vi "TestExec.Send Funct RTN Data.vi"(8 "Error":errorcluster, 9 "RTN Route (Data2)":variant, 10 "RTN Data":T1 {"MeasData"."Status" items=["LOG", "PASS", "FAIL", "ERROR"]; "Attr"."Status" items=["LOG", "PASS", "FAIL", "ERROR"]; "Num"."Status" items=["LOG", "PASS", "FAIL", "ERROR"]}, 11 "Q In":refnum<queue>) -> (0 "error out":errorcluster)   [LabVIEW 2018]
uses:
  <vilib>/KATE/Queues/Q.Element.ctl
  TestExec.Local Result Data.ctl
  Results/Result.Attribute.ctl
  Results/Result.Measurement and Attribute Item Status.ctl
  Results/Result.Numeric.ctl
  Results/Result.Limit Type.ctl
  Results/Result XML/TestResult.SW Item.ctl
  Reports/Report.Result FileDataObject.ctl
  Results/Result.Measurement Item.ctl
  <vilib>/KATE/Queues/Queue Utils.lvlib
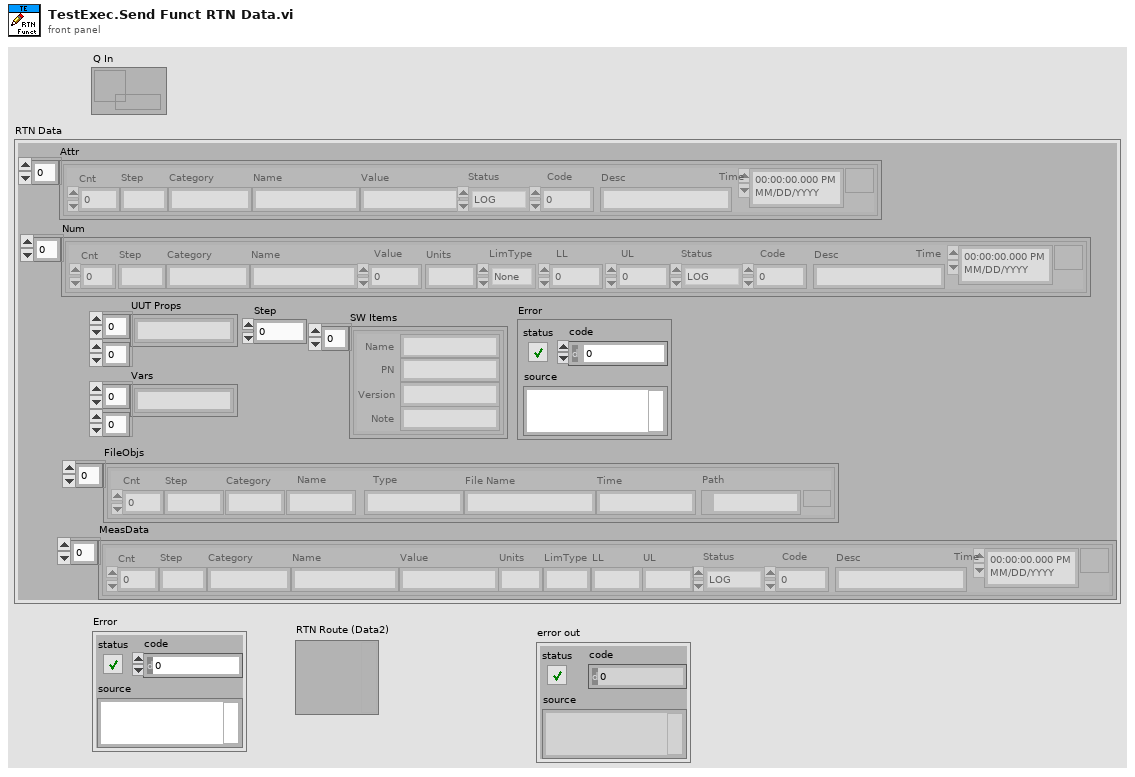
[diagram p1: front panel]
types:
  T1 = typedef "TestExec.Local Result Data.ctl" = cluster{"Attr":T2[], "Num":T4[], "UUT Props":string[][], "Vars":string[][], "SW Items":T6[], "Error":errorcluster, "Step":i32, "FileObjs":T7[], "MeasData":T8[]}
  T2 = typedef "Result.Attribute.ctl" = cluster{"Cnt":i32, "Step":string, "Category":string, "Name":string, "Value":string, "Status":T3, "Code":i32, "Desc":string, "Time":timestamp}
  T3 = typedef "Result.Measurement and Attribute Item Status.ctl" = i32
  T4 = typedef "Result.Numeric.ctl" = cluster{"Cnt":i32, "Step":string, "Category":string, "Name":string, "Value":dbl, "Units":string, "LimType":T5, "LL":dbl, "UL":dbl, "Status":T3, "Code":i32, "Desc":string, "Time":timestamp}
  T5 = typedef "Result.Limit Type.ctl" = enum16{"None", "EQ", "NE", "GT", "LT", "GE", "LE", "GTLT", "GELE", "GELT", "GTLE", "LTGT", "LEGE", "LEGT", "LTGE", "Contains", "NotContains"}
  T6 = typedef "TestResult.SW Item.ctl" = cluster{"Name":string, "PN":string, "Version":string, "Note":string}
  T7 = typedef "Report.Result FileDataObject.ctl" = cluster{"Cnt":i32, "Step":string, "Category":string, "Name":string, "Type":string, "File Name":string, "Time":string, "Path":path}
  T8 = typedef "Result.Measurement Item.ctl" = cluster{"Cnt":i32, "Step":string, "Category":string, "Name":string, "Value":string, "Units":string, "LimType":string, "LL":string, "UL":string, "Status":T3, "Code":i32, "Desc":string, "Time":timestamp}
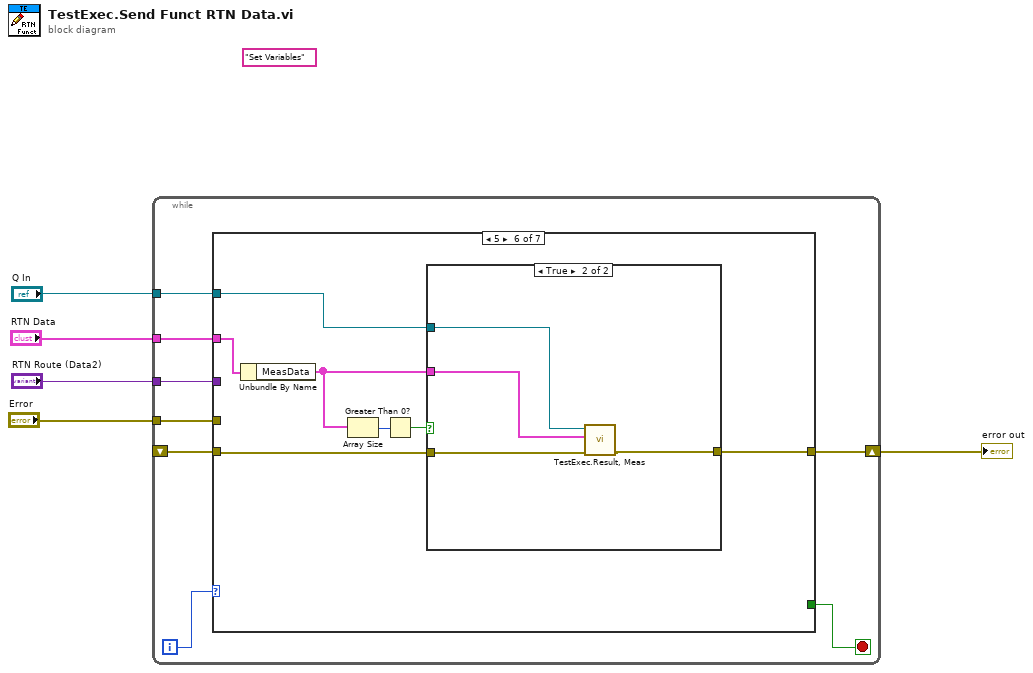
[diagram p0: block diagram]
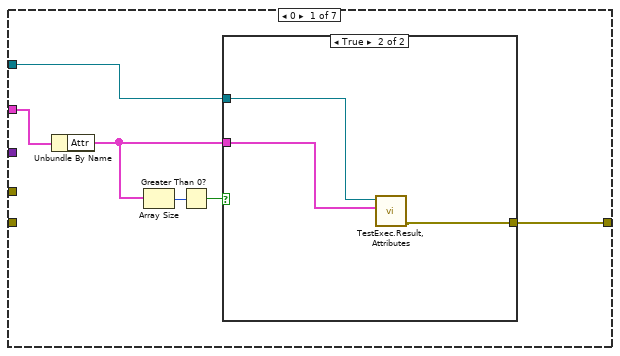
[diagram p2: hidden frame]
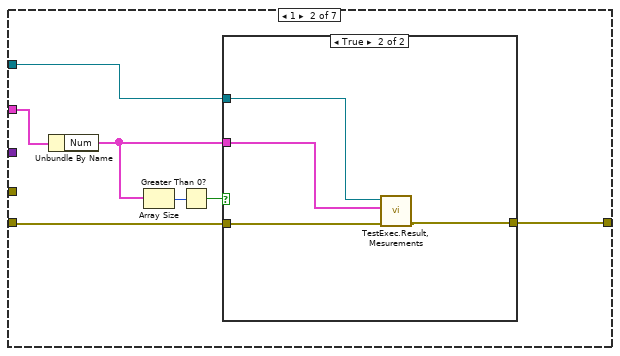
[diagram p4: hidden frame]
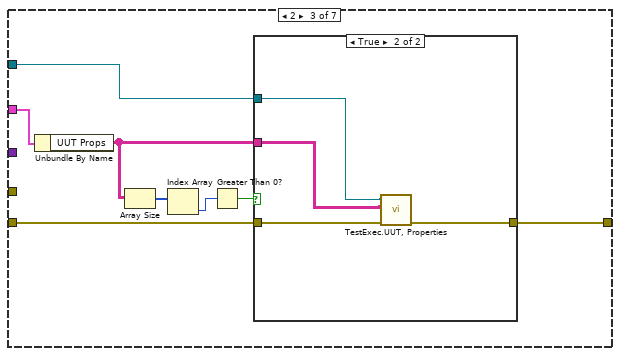
[diagram p6: hidden frame]
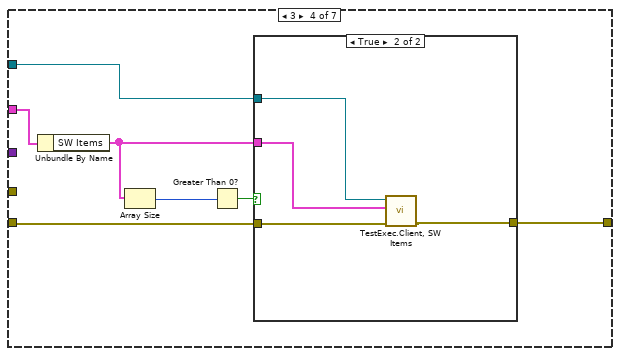
[diagram p8: hidden frame]
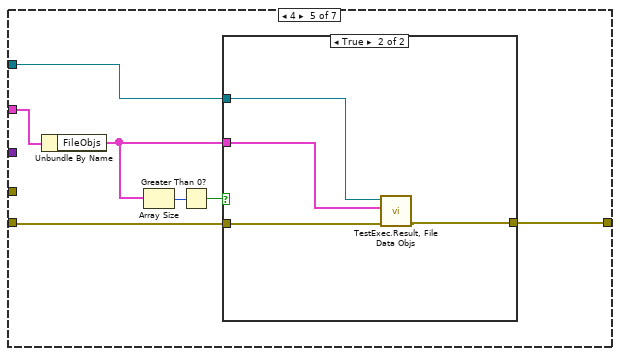
[diagram p10: hidden frame]
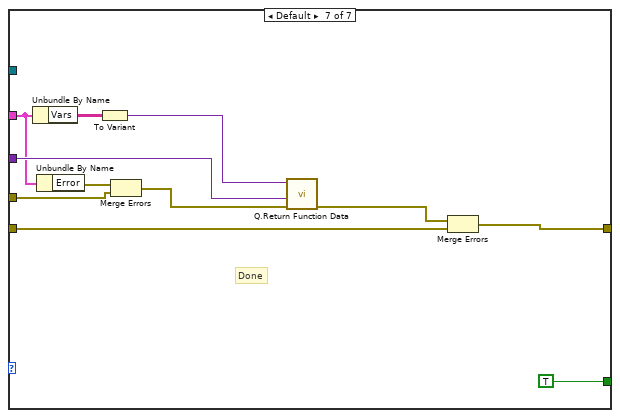
[diagram p13: hidden frame]
diagram:
  (unwired) "Set Variables" ("Cmd")
  n1 = while {
    shift-right: [w10] -> w5
    shift-left: _ -> [w11]
    tunnel: "RTN Data" -> [w9]
    tunnel: "Q In" -> [w8]
    tunnel: "RTN Route (Data2)" -> [w7]
    tunnel: "Error" -> [w6]
    i -> [w13]
    stop <- w12 stop-if-true
    n2 = case shown="5" w13 {
      tunnel: [_ _ _ _ _ _ TRUE] -> w12
      tunnel: w11 -> [_ w23 w34 w46 w57 w68 w84]
      tunnel: [w15 w25 w38 w49 w59 w70 w83] -> w10
      tunnel: w9 -> [w19 w29 w41 w52 w63 w74 w82]
      tunnel: w8 -> [w14 w24 w37 w48 w58 w69 _]
      tunnel: w7 -> [_ _ _ _ _ _ w88]
      tunnel: w6 -> [_ _ _ _ _ _ w80]
      frame 0 {
        n3 = Unbundle By Name(w19) -> ("Attr"=w16:T2[])
        n4 = Array Size(array=w16) -> (size(s)=w17:i32)
        n5 = Greater Than 0?(x=w17) -> (x > 0?=w18:bool)
        n6 = case shown="True" w18 {
          tunnel: w16 -> [_ w21]
          tunnel: [_ w20] -> w15
          tunnel: w14 -> [_ w22]
          frame False {
          }
          frame True {
            n7 = call "TestExec.Result, Attributes.vi"("Attributes"=w21, "Q In"=w22) -> ("error out"=w20:errorcluster)  [unwired: 9 in]
          }
        }
      }
      frame 1 {
        n8 = Unbundle By Name(w29) -> ("Num"=w26:T4[])
        n9 = Array Size(array=w26) -> (size(s)=w27:i32)
        n10 = Greater Than 0?(x=w27) -> (x > 0?=w28:bool)
        n11 = case shown="True" w28 {
          tunnel: w26 -> [_ w32]
          tunnel: [_ w31] -> w25
          tunnel: w24 -> [_ w33]
          tunnel: w23 -> [_ w30]
          frame False {
          }
          frame True {
            n12 = call "TestExec.Result, Mesurements.vi"("error in"=w30, "Measurements"=w32, "Q In"=w33) -> ("error out"=w31:errorcluster)  [unwired: 8 in]
          }
        }
      }
      frame 2 {
        n13 = Unbundle By Name(w41) -> ("UUT Props"=w39:string[][])
        n14 = Array Size(array=w39) -> (size(s)=w36:i32[])
        n15 = Index Array(array=w36) -> (element=w35:i32)  [unwired: 1 in]
        n16 = Greater Than 0?(x=w35) -> (x > 0?=w40:bool)
        n17 = case shown="True" w40 {
          tunnel: w39 -> [_ w44]
          tunnel: [_ w43] -> w38
          tunnel: w37 -> [_ w45]
          tunnel: w34 -> [_ w42]
          frame False {
          }
          frame True {
            n18 = call "TestExec.UUT, Properties.vi"("error in"=w42, "UUT Properties"=w44, "Q In"=w45) -> ("error out"=w43:errorcluster)  [unwired: 8 in]
          }
        }
      }
      frame 3 {
        n19 = Unbundle By Name(w52) -> ("SW Items"=w50:T6[])
        n20 = Array Size(array=w50) -> (size(s)=w47:i32)
        n21 = Greater Than 0?(x=w47) -> (x > 0?=w51:bool)
        n22 = case shown="True" w51 {
          tunnel: w50 -> [_ w54]
          tunnel: [_ w55] -> w49
          tunnel: w48 -> [_ w56]
          tunnel: w46 -> [_ w53]
          frame False {
          }
          frame True {
            n23 = call "TestExec.Client, SW Items.vi"("error in"=w53, "SW Items"=w54, "Q In"=w56) -> ("error out"=w55:errorcluster)  [unwired: 7 in, 1 out]
          }
        }
      }
      frame 4 {
        n24 = Unbundle By Name(w63) -> ("FileObjs"=w60:T7[])
        n25 = Array Size(array=w60) -> (size(s)=w61:i32)
        n26 = Greater Than 0?(x=w61) -> (x > 0?=w62:bool)
        n27 = case shown="True" w62 {
          tunnel: w60 -> [_ w66]
          tunnel: [_ w65] -> w59
          tunnel: w58 -> [_ w67]
          tunnel: w57 -> [_ w64]
          frame False {
          }
          frame True {
            n28 = call "TestExec.Result, File Data Objs.vi"("error in"=w64, "File Data Objs"=w66, "Q In"=w67) -> ("error out"=w65:errorcluster)  [unwired: 8 in]
          }
        }
      }
      frame 5 {
        n29 = Unbundle By Name(w74) -> ("MeasData"=w71:T8[])
        n30 = Array Size(array=w71) -> (size(s)=w72:i32)
        n31 = Greater Than 0?(x=w72) -> (x > 0?=w73:bool)
        n32 = case shown="True" w73 {
          tunnel: w71 -> [_ w77]
          tunnel: [_ w76] -> w70
          tunnel: w69 -> [_ w78]
          tunnel: w68 -> [_ w75]
          frame False {
          }
          frame True {
            n33 = call "TestExec.Result, Meas.vi"("error in"=w75, "Meas"=w77, "Q In"=w78) -> ("error out"=w76:errorcluster)  [unwired: 8 in]
          }
        }
      }
      frame Default {
        # "Done"
        n34 = Unbundle By Name(w82) -> ("Vars"=w87:string[][])
        n35 = Unbundle By Name(w82) -> ("Error"=w81:errorcluster)
        n36 = To Variant(anything=w87) -> (Variant=w86:variant)
        n37 = Merge Errors(w81, w80) -> (w79:errorcluster)
        n38 = call <vilib>:"Q.Return Function Data.vi"("error in"=w79, "Data2"=w88, "Ret Data"=w86) -> ("error out"=w85:errorcluster)  [unwired: 8 in]
        n39 = Merge Errors(w85, w84) -> (w83:errorcluster)
      }
    }
  }
  "error out" <- w5
